vi "WriteToXMLAzElParam.vi"(8 "error in (no error)":errorcluster, 10 "Class Label":string="AzElParameters") -> (0 "error out":errorcluster, 2 "XML out":string="<>\n  <azimuth>\n    <degreesArc>0</degreesArc>\n    <minutesArc>0</minutesArc>\n    <secondsArc>0</secondsArc>\n  </azimuth>\n  <elevation>\n    <degreesAlt>90</degreesAlt>\n    <minutesArc>0</minutesArc>\n    <secondsArc>0</secondsArc>\n  </elevation>\n</>")   [LabVIEW 2012]
uses:
  <userlib>/Common/XML/XMLParser/XMLParser.lvclass
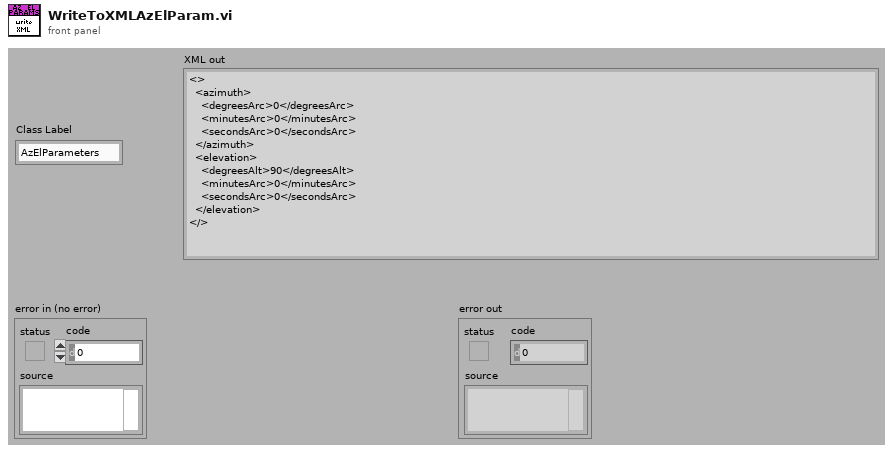
[diagram p1: front panel]
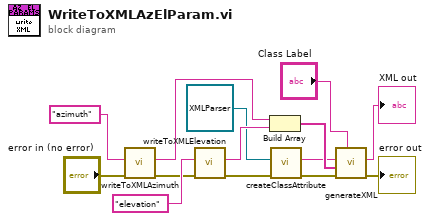
[diagram p0: block diagram]
diagram:
  n1 = call <userlib>:"writeToXMLAzimuth.vi"("error in (no error)"="error in (no error)", "Class Label"="azimuth") -> ("error out"=w9:errorcluster, "XML out"=w7:string)  [unwired: 8 in]
  n2 = call <userlib>:"writeToXMLElevation.vi"("error in (no error)"=w9, "Class Label"="elevation") -> ("error out"=w4:errorcluster, "XML out"=w6:string)  [unwired: 8 in]
  n3 = Build Array(w7, w6) -> (w5:string[])
  n4 = call <userlib>:"createClassAttribute.vi"("error in (no error)"=w4, "LVClass In"=refnum<class "XMLParser.lvclass"> refnum ("XMLParser.lvclass")) -> ("error out"=w3:errorcluster, "AttributeString"=w2:string)  [unwired: 7 in, 1 out]
  n5 = call <userlib>:"generateXML.vi"("elementName"="Class Label", "error in"=w3, "childrenXML"=w5, "attributeString"=w2) -> ("error out"=→"error out":errorcluster, "XML out"=→"XML out":string)  [unwired: 5 in, 1 out]
